vi "SRV_Launch Sensor View Tab GUI.vi"(0 "VI Path":path, 5 "Sensors Config File Path":path, 7 "SRV In":refnum<k5>, 9 "Vista or Later?":bool, 11 "error in (no error)":errorcluster, 12 "Main Controller ref":refnum<vi>, 13 "Expand-Collapse":bool) -> (4 "VI refnum out":refnum<vi>, 8 "resulting string":string, 15 "error out":errorcluster)   [LabVIEW 2014]
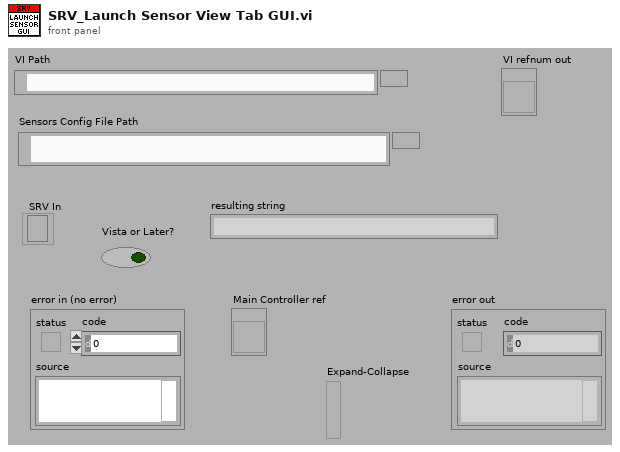
[diagram p1: front panel]
types:
  T1 = enum32{"Bad", "Idle", "Run top level", "Running"}
  T2 = enum32{"Invalid", "Standard", "Closed", "Hidden", "Minimized", "Maximized"}
  T3 = enum32{"Invalid", "Default", "Floating", "Floating/Auto-Hide", "Modal"}
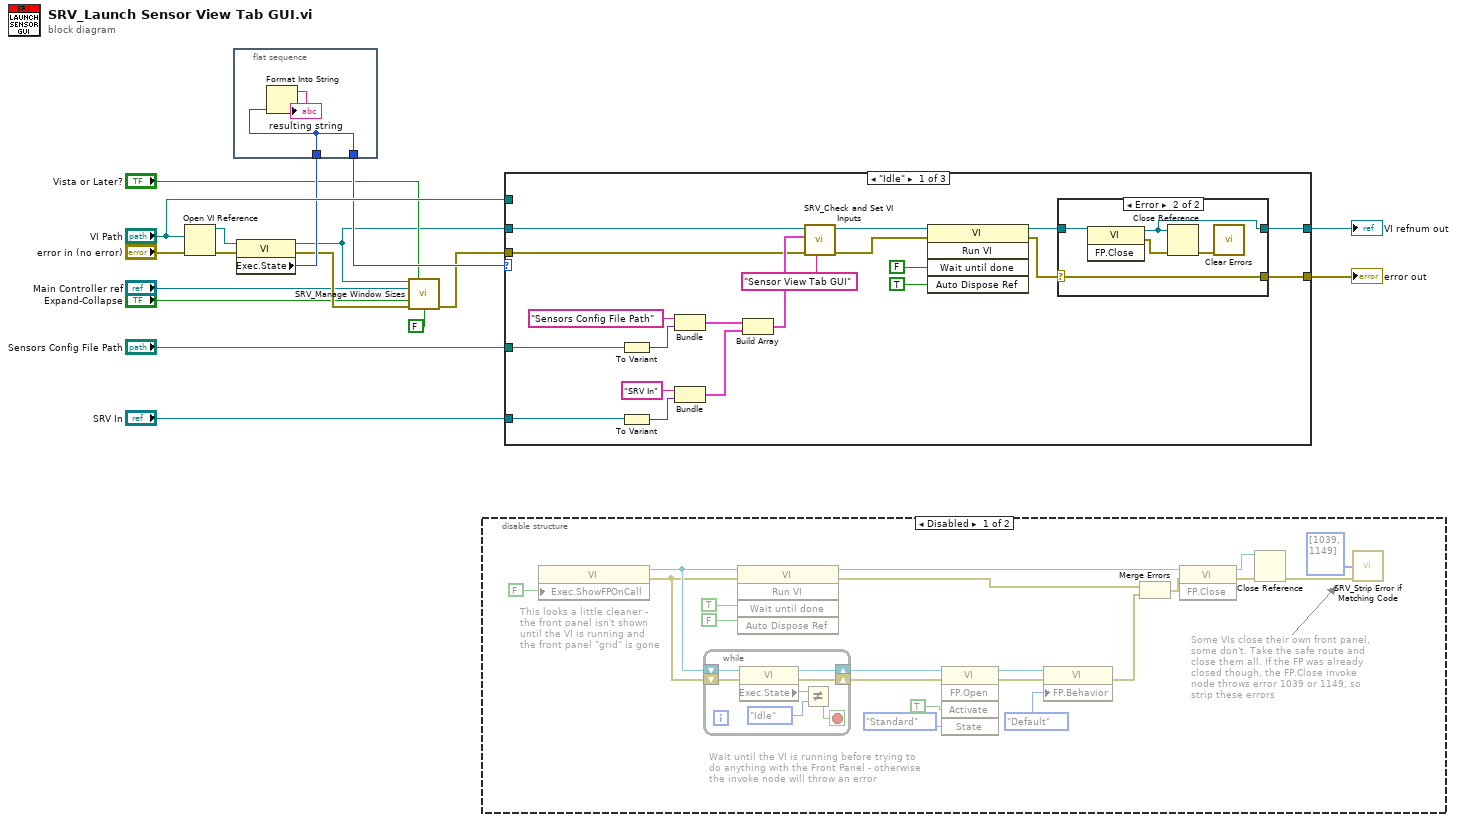
[diagram p0: block diagram]
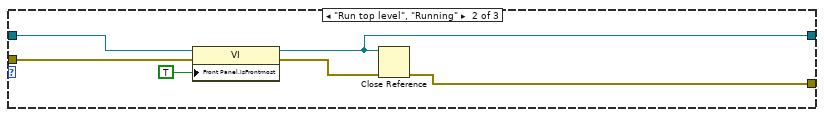
[diagram p3: hidden frame]
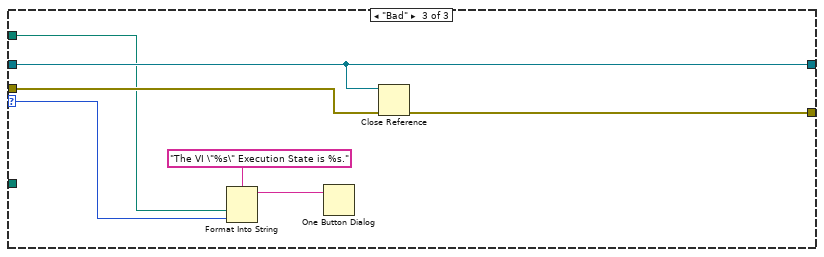
[diagram p4: hidden frame]
diagram:
  n1 = Open VI Reference(vi path="VI Path", error in (no error)="error in (no error)") -> (vi reference=w12:refnum<vi>, error out=w11:errorcluster)  [unwired: 4 out]
  n2 = flat-sequence {
    tunnel: w9 -> [w18]
    tunnel: [w18] -> w8
    frame #0 {
      n3 = Format Into String(w18) -> (resulting string=→"resulting string":string)  [unwired: 3 in, 1 out]
    }
  }
  n4 = property class="VI"(reference=w12, error in=w11) -> (reference out=w4:refnum<vi>, error out=w7:errorcluster, "Exec.State"=w9:T1)
  n5 = call "SRV_Manage Window Sizes.vi"("Sensor View ref"=w4, "Vista or Later?"="Vista or Later?", "Main Controller ref"="Main Controller ref", "Expand-Collapse"="Expand-Collapse", "error in (no error)"=w7, "Update Main Controller Window Size (T)"=FALSE) -> ("error out"=w6:errorcluster)  [unwired: 9 in]
  n6 = disable-structure shown="Disabled" {
    frame Disabled {
      # "Wait until the VI is running before trying to\ndo anything with the Front Panel - otherwise\nthe invoke node will throw an error"
      # "This looks a little cleaner -\nthe front panel isn't shown\nuntil the VI is running and\nthe front panel \"grid\" is gone"
      # "Some VIs close their own front panel,\nsome don't. Take the safe route and\nclose them all. If the FP was already\nclosed though, the FP.Close invoke\nnode throws error 1039 or 1149, so \nstrip these errors"
      n7 = property class="VI"("Exec.ShowFPOnCall"=FALSE ("Execution:Show Front Panel On Call")) -> (reference=w37:refnum<vi>, reference out=w38:refnum<vi>, error in=w35:errorcluster, error out=w36:errorcluster)
      n8 = while {
        shift-right: [w43] -> w28
        shift-left: w38 -> [w48]
        shift-right: [w42] -> w29
        shift-left: w36 -> [w47]
        stop <- w44 stop-if-true
        n9 = property class="VI"(reference=w48, error in=w47) -> (reference out=w43:refnum<vi>, error out=w42:errorcluster, "Exec.State"=w46:T1)
        n10 = Not Equal?(x=w46, y=T1."Idle") -> (x != y?=w44:bool)
      }
      n11 = invoke class="VI" method="Run VI"(reference=w38, error in=w36, "Wait until done"=TRUE ("Activate"), "Auto Dispose Ref"=FALSE ("Activate")) -> (reference out=w22:refnum<vi>, error out=w34:errorcluster)  [unwired: 1 in, 3 out]
      n12 = invoke class="VI" method="FP.Open"(reference=w28, error in=w29, "Activate"=TRUE, "State"=T2."Standard") -> (reference out=w30:refnum<vi>, error out=w31:errorcluster)  [unwired: 1 in, 3 out]
      n13 = property class="VI"(reference=w30, error in=w31, "FP.Behavior"=T3."Default" ("Front Panel Window:Behavior")) -> (error out=w33:errorcluster)  [unwired: 1 out]
      n14 = Merge Errors(w34, w33) -> (w32:errorcluster)
      n15 = invoke class="VI" method="FP.Close"(reference=w22, error in=w32) -> (reference out=w24:refnum<vi>, error out=w23:errorcluster)  [unwired: 1 in, 1 out]
      n16 = Close Reference(reference=w24, error in (no error)=w23) -> (error out=w40:errorcluster)
      n17 = call "SRV_Strip Error if Matching Code.vi"("error in (no error)"=w40, "Strip Codes"=i32[] [1039, 1149]) -> ()  [unwired: 8 in, 1 out]
    }
    frame Enabled {
    }
  }
  n18 = case shown="\"Idle\"" w8 {
    selector: w8 -> [_ _ w83]
    tunnel: "Sensors Config File Path" -> [w60 _ _]
    tunnel: "SRV In" -> [w56 _ _]
    tunnel: [w54 w81 w87] -> w14
    tunnel: [w52 w78 w88] -> w13
    tunnel: w4 -> [w50 w79 w88]
    tunnel: w6 -> [w49 w77 w86]
    tunnel: "VI Path" -> [_ _ w82]
    frame "Idle" {
      n19 = To Variant(anything=w60) -> (Variant=w61:variant)
      n20 = To Variant(anything=w56) -> (Variant=w59:variant)
      n21 = Bundle("Sensors Config File Path", "Variant"=w61) -> (w64:cluster{string, "Variant":variant})  [unwired: 1 in]
      n22 = Bundle("SRV In", "Variant"=w59) -> (w57:cluster{string, "Variant":variant})  [unwired: 1 in]
      n23 = Build Array(w64, w57) -> (w62:cluster{string, "Variant":variant}[])
      n24 = call "SRV_Check and Set VI Inputs.vi"("Callback Identifier"="Sensor View Tab GUI", "error in (no error)"=w49, "Required Controls"=w62, "VI Refnum In"=w50) -> ("error out"=w66:errorcluster, "VI Refnum Out"=w65:refnum<vi>)  [unwired: 6 in]
      n25 = invoke class="VI" method="Run VI"(reference=w65, error in=w66, "Wait until done"=FALSE, "Auto Dispose Ref"=TRUE ("Auto Dispose Reference")) -> (reference out=w53:refnum<vi>, error out=w55:errorcluster)  [unwired: 1 in, 3 out]
      n26 = case shown="Error" w55 {
        selector: w55 -> [w70 w72]
        tunnel: w53 -> [w69 w74]
        tunnel: [w70 w72] -> w54
        tunnel: [w69 w71] -> w52
        frame No Error {
        }
        frame Error {
          n27 = invoke class="VI" method="FP.Close"(reference=w74) -> (reference out=w71:refnum<vi>, error out=w73:errorcluster)  [unwired: 2 in, 1 out]
          n28 = Close Reference(reference=w71, error in (no error)=w73) -> (error out=w75:errorcluster)
          n29 = call <vilib>:"Clear Errors.vi"("error in (no error)"=w75) -> ()  [unwired: 5 in, 2 out]
        }
      }
    }
    frame "Run top level", "Running" {
      n30 = property class="VI"(reference=w79, error in=w77, "Front Panel.IsFrontmost"=TRUE ("Front Panel Window:Is Frontmost")) -> (reference out=w78:refnum<vi>, error out=w76:errorcluster)
      n31 = Close Reference(reference=w78, error in (no error)=w76) -> (error out=w81:errorcluster)
    }
    frame "Bad" {
      n32 = Format Into String(format string="The VI \"%s\" Execution State is %s.", w82, w83) -> (resulting string=w84:string)  [unwired: 2 in, 1 out]
      n33 = One Button Dialog(message=w84) -> ()  [unwired: 1 in, 1 out]
      n34 = Close Reference(reference=w88, error in (no error)=w86) -> (error out=w87:errorcluster)
    }
  }
  "error out" <- w14
  "VI refnum out" <- w13
